vi "Actor Core.vi"(8 "error in":errorcluster, 11 "Nested in":refnum<class "TriaxesStageController.lvclass">) -> (0 "error out":errorcluster, 3 "Actor out":refnum<class "Actor.lvclass">)   [LabVIEW 2020, in "TriaxesStageController.lvlib" / "TriaxesStageController.lvclass"]
doc: "(<B>Filename</B>: Actor Framework.lvlib:Actor.lvclass:Actor Core.vi)\n\nReceives messages to the actor, reacts to them, and initiates any error handling that may shut the actor down.\n\nDescendant classes may override this VI to append parallel tasks for the actor to complete while it handles messages. Overrides use the Call Parent Method node."
uses:
  TriaxesStageController.lvclass
  C:/Program Files/National Instruments/LabVIEW 2020/vi.lib/ActorFramework/Actor/Actor.lvclass
  <vilib>/ActorFramework/Actor/Actor.lvclass
  TriaxesStageController.lvclass/TriaxesStageController.ctl
  <vilib>/ActorFramework/Actor/Actor.lvclass/Actor.ctl
  <vilib>/ActorFramework/Message Enqueuer/Message Enqueuer.lvclass/Message Enqueuer.ctl
  Model/Hardware Abstraction Layer/Component/Stage/Stage Messages/SetRelativePositionUm Msg/SetRelativePositionUm Msg.lvclass/SetRelativePositionUm Msg.ctl
  Model/Hardware Abstraction Layer/Component/Stage/Stage Messages/SetPositionUm Msg/SetPositionUm Msg.lvclass/SetPositionUm Msg.ctl
  Model/Hardware Abstraction Layer/Component/Device/Device Messages/SetSamplingRate Msg/SetSamplingRate Msg.lvclass/SetSamplingRate Msg.ctl
  <vilib>/ActorFramework/Message Enqueuer/Init from Existing Queue.vi
  <vilib>/ActorFramework/Message Enqueuer/Enqueue.vi
  Model/Hardware Abstraction Layer/Component/Stage/Stage Messages/SetRelativePositionUm Msg/SetRelativePositionUm Msg.lvclass
  C:/Program Files/National Instruments/LabVIEW 2020/vi.lib/ActorFramework/Message/Message.lvclass
  Model/Hardware Abstraction Layer/Component/Stage/Stage Messages/SetPositionUm Msg/SetPositionUm Msg.lvclass
  Model/Hardware Abstraction Layer/Component/Device/Device Messages/SetSamplingRate Msg/SetSamplingRate Msg.lvclass
  <vilib>/ActorFramework/Stop Msg/Stop Msg.lvclass
  <vilib>/ActorFramework/Message Priority Queue/Priority Enqueue.vi
  <vilib>/ActorFramework/Message Enqueuer/Message Enqueuer.lvclass
panel:
  in  "SamplingRate(Hz)":dbl min=0.0 max=200.0
  in  "Stop Button":bool
  in  "StageZ":dbl min=0.0 max=200.0
  in  "StageY":dbl min=0.0 max=200.0
  in  "StageX":dbl min=0.0 max=200.0
  out "NanoStage X":dbl(graph)
  out "NanoStage  Y":dbl(graph)
  out "NanoStage Z":dbl(graph)
  in  "ZIncreatement+":dbl min=0.0 max=50.0
  in  "ZIncreatement++":dbl min=0.0 max=50.0
  in  "StageX-":bool
  in  "StageX+":bool
  in  "StageY+":bool
  in  "StageY-":bool
  in  "StageY++":bool
  in  "StageX--":bool
  in  "StageX++":bool
  in  "StageY--":bool
  in  "XYIncreatement+":dbl min=0.0 max=50.0
  in  "XYIncreatement++":dbl min=0.0 max=100.0
  in  "StageZ++":bool
  in  "StageZ--":bool
  in  "StageZ+":bool
  in  "StageZ-":bool
  # "Increment(um)"
  # "um"
  # "um"
  # "um"
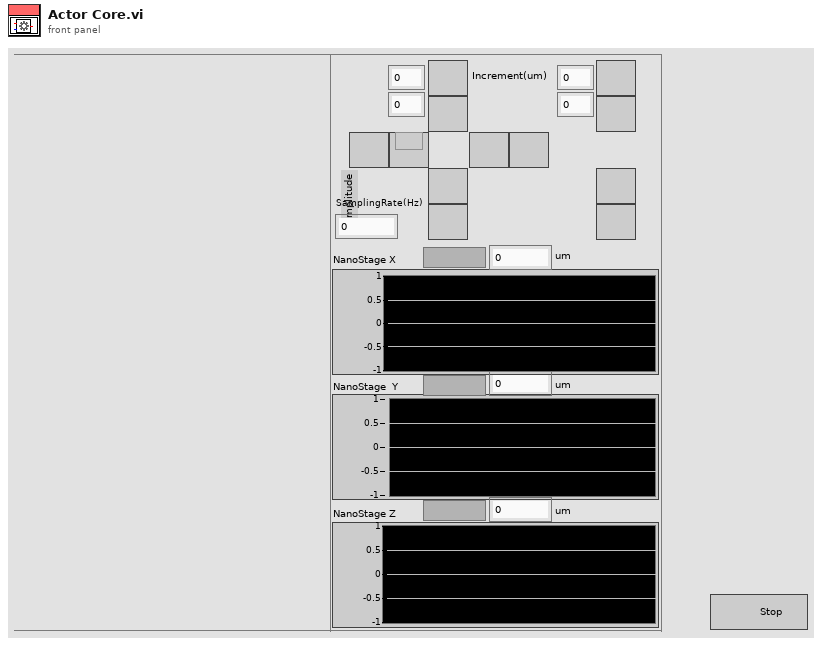
[diagram p1: front panel]
types:
  T1 = cluster{"Stop":refnum<user-event>, "NanoStage X":refnum<user-event>, "NanoStage  Y":refnum<user-event>, "NanoStage Z":refnum<user-event>}
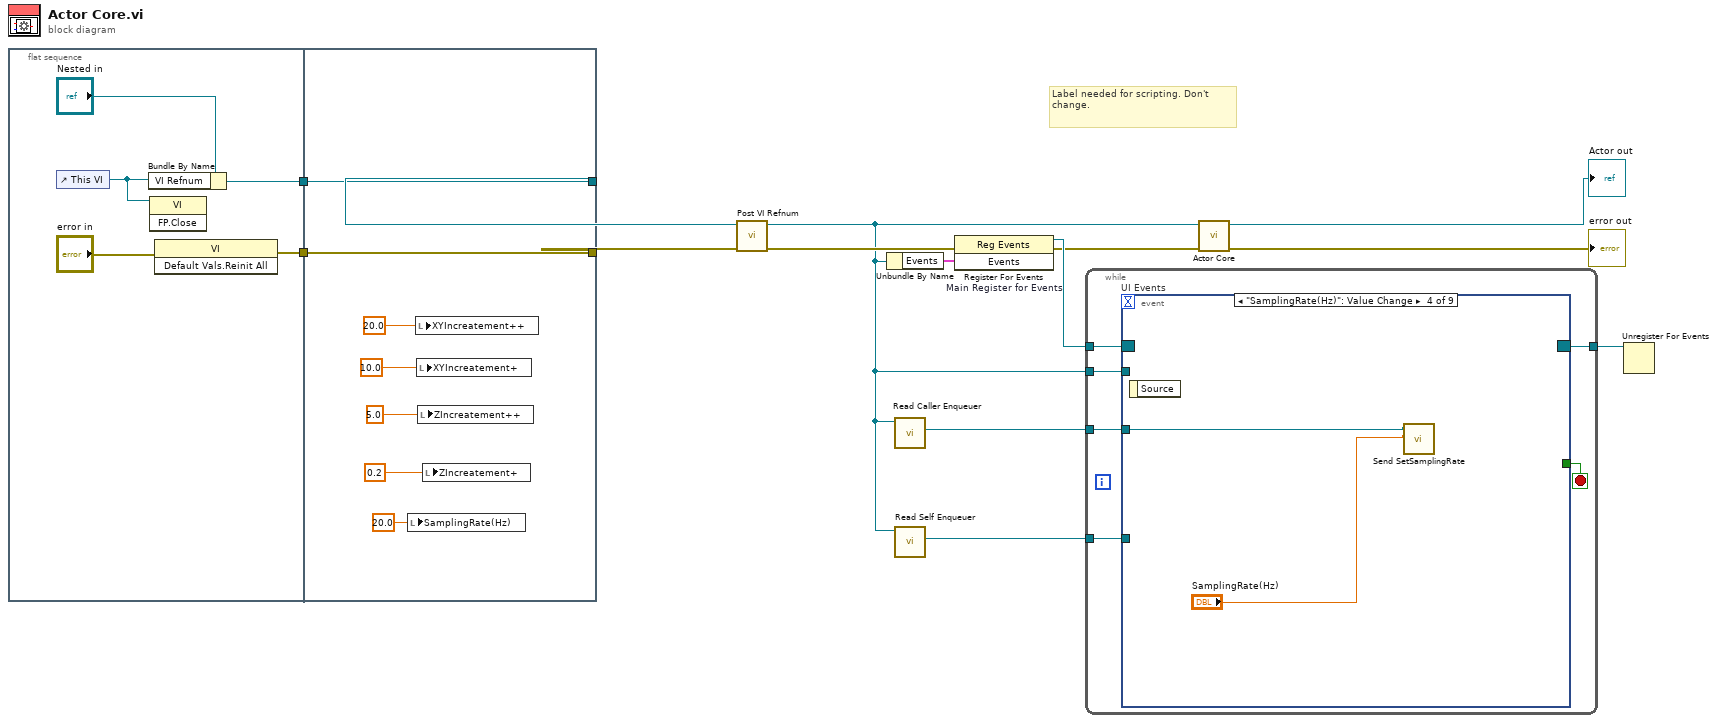
[diagram p0: block diagram]
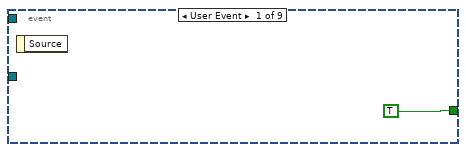
[diagram p2: hidden frame]
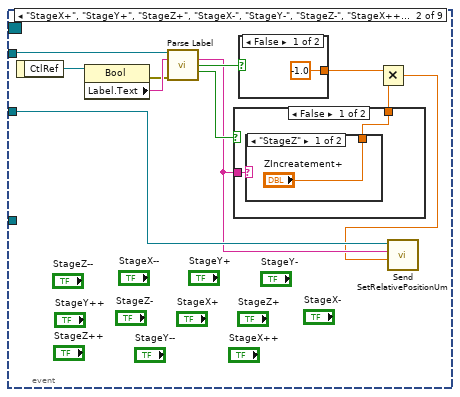
[diagram p3: hidden frame]
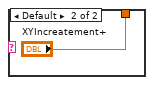
[diagram p4: hidden frame]
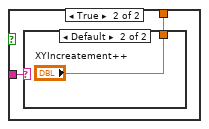
[diagram p5: hidden frame]
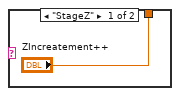
[diagram p6: hidden frame]
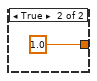
[diagram p7: hidden frame]
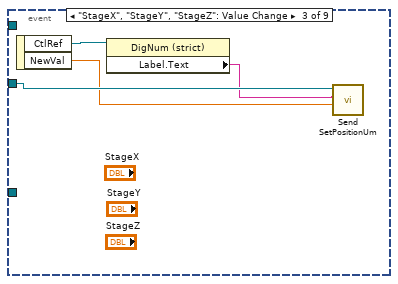
[diagram p8: hidden frame]
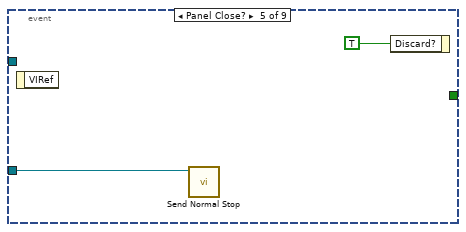
[diagram p9: hidden frame]
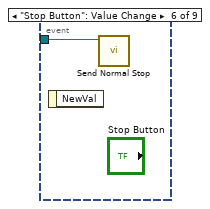
[diagram p10: hidden frame]
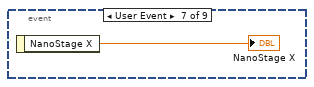
[diagram p11: hidden frame]
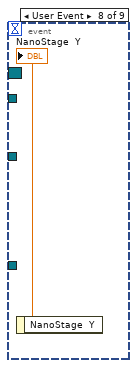
[diagram p12: hidden frame]
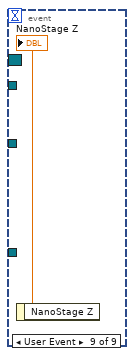
[diagram p13: hidden frame]
diagram:
  # "Label needed for scripting. Don't change."
  n1 = flat-sequence {
    tunnel: [w17] -> w2
    tunnel: [w16] -> w1
    tunnel: [w25] -> w6
    tunnel: [w26] -> w7
    tunnel: w2 -> [w26]
    tunnel: w1 -> [w25]
    frame #0 {
      n2 = control-ref of="This VI"() -> (w15:refnum<vi>)
      n3 = Bundle By Name(cluster="Nested in", "VI Refnum"=w15) -> (w17:refnum<class "TriaxesStageController.lvclass">)
      n4 = invoke class="VI" method="FP.Close"(reference=w15) -> ()  [unwired: 2 in, 3 out]
      n5 = invoke class="VI" method="Default Vals.Reinit All"(error in="error in") -> (error out=w16:errorcluster)  [unwired: 2 in, 2 out]
    }
    frame #1 {
      n6 = local write "SamplingRate(Hz)"(20.0 ("Interval(ms)")) -> ()
      n7 = local write "XYIncreatement++"(20.0 ("XYIncreatement++")) -> ()
      n8 = local write "XYIncreatement+"(10.0 ("XYIncreatement++")) -> ()
      n9 = local write "ZIncreatement++"(5.0 ("XYIncreatement++")) -> ()
      n10 = local write "ZIncreatement+"(0.2 ("XYIncreatement++")) -> ()
    }
  }
  n11 = call-dynamic "Post VI Refnum.vi"("error in (no error)"=w6, "Stage Controller in"=w7) -> ("error out"=w5:errorcluster, "Stage Controller out"=w4:refnum<class "TriaxesStageController.lvclass">)  [unwired: 8 in]
  n12 = Unbundle By Name(w4) -> ("Events"=w11:T1)
  n13 = call <vilib>:"Read Caller Enqueuer.vi"("Actor"=w4) -> ("Caller Enqueuer"=w3:refnum<class "Message Enqueuer.lvclass">)  [unwired: 10 in]
  n14 = call <vilib>:"Read Self Enqueuer.vi"("Actor"=w4) -> ("Self Enqueuer"=w9:refnum<class "Message Enqueuer.lvclass">)  [unwired: 10 in]
  n15 = register-events "Main Register for Events"(error in=w5, w11) -> (reference out=w12:refnum<event-registration>, error out=w8:errorcluster)  [unwired: 1 in]
  n16 = while {
    tunnel: w12 -> [w32]
    tunnel: [w30] -> w10
    tunnel: w9 -> [w29]
    tunnel: w4 -> [w28]
    tunnel: w3 -> [w27]
    stop <- w31 stop-if-true
    n17 = event "UI Events" shown="[3] \"SamplingRate(Hz)\": Value Change" {
      selector: w32 -> [_ _ _ _ _ _ _ _ _]
      dyn-events: [_ _ _ _ _ _ _ _ _] -> w30
      timeout: _ -> [_ _ _ _ _ _ _ _ _]
      tunnel: [TRUE _ _ _ _ _ _ _ _] -> w31
      tunnel: w29 -> [_ _ _ _ w61 w63 _ _ _]
      tunnel: w28 -> [_ w41 _ _ _ _ _ _ _]
      tunnel: w27 -> [_ w36 w57 w60 _ _ _ _ _]
      event User Event {
        n18 = event-data() -> ()  [unwired: 1 in, 1 out]
      }
      event "StageX+", "StageY+", "StageZ+", "StageX-", "StageY-", "StageZ-", "StageX++", "StageY++", "StageZ++", "StageX--", "StageY--", "StageZ--": Value Change {
        n19 = event-data() -> ("CtlRef"=w44:refnum<vi>)  [unwired: 1 in]
        n20 = property class="Bool"(reference=w44) -> (error out=w42:errorcluster, "Label.Text"=w43:string)  [unwired: 1 in, 1 out]
        n21 = call-dynamic "Parse Label.vi"("Stage Controller in"=w41, "Label.Text"=w43, "error in (no error)"=w42) -> ("Stage Label"=w35:string, "Increase?"=w40:bool, "Big Step?"=w39:bool)  [unwired: 8 in, 2 out]
        n22 = case shown="False" w39 {
          tunnel: [w46 w50] -> w37
          tunnel: w35 -> [w45 w49]
          frame False {
            n23 = case shown="\"StageZ\"" w45 {
              tunnel: ["ZIncreatement+" "XYIncreatement+"] -> w46
              frame "StageZ" {
              }
              frame Default {
              }
            }
          }
          frame True {
            n24 = case shown="Default" w49 {
              tunnel: ["ZIncreatement++" "XYIncreatement++"] -> w50
              frame "StageZ" {
              }
              frame Default {
              }
            }
          }
        }
        n25 = case shown="False" w40 {
          tunnel: [-1.0 ("XYIncreatement+") 1.0 ("XYIncreatement+")] -> w38
          frame False {
          }
          frame True {
          }
        }
        n26 = Multiply(x=w38, y=w37) -> (x*y=w34:dbl)
        n27 = call "Send SetRelativePositionUm.vi"("RelativeMoveum"=w34, "Stage Label"=w35, "Message Enqueuer"=w36) -> ()  [unwired: 7 in, 2 out]
      }
      event "StageX", "StageY", "StageZ": Value Change {
        n28 = event-data() -> ("CtlRef"=w58:refnum<vi>, "NewVal"=w55:dbl)  [unwired: 1 in]
        n29 = property class="DigNum (strict)"(reference=w58) -> ("Label.Text"=w56:string)  [unwired: 1 in, 2 out]
        n30 = call "Send SetPositionUm.vi"("Positionum"=w55, "Stage Label"=w56, "Message Enqueuer"=w57) -> ()  [unwired: 7 in, 2 out]
      }
      event "SamplingRate(Hz)": Value Change {
        n31 = event-data() -> ()  [unwired: 1 in, 1 out]
        n32 = call "Send SetSamplingRate.vi"("SamplingRate"="SamplingRate(Hz)", "Message Enqueuer"=w60) -> ()  [unwired: 8 in, 2 out]
      }
      event Panel Close? {
        n33 = event-data() -> ()  [unwired: 1 in, 1 out]
        n34 = call <vilib>:"Send Normal Stop.vi"("Message Enqueuer"=w61) -> ()  [unwired: 10 in, 1 out]
        n35 = event-data("Discard?"=TRUE) -> ()  [unwired: 1 in, 1 out]
      }
      event "Stop Button": Value Change {
        n36 = event-data() -> ()  [unwired: 1 in, 1 out]
        n37 = call <vilib>:"Send Normal Stop.vi"("Message Enqueuer"=w63) -> ()  [unwired: 10 in, 1 out]
      }
      event User Event {
        n38 = event-data() -> ("NanoStage X"=→"NanoStage X":dbl)  [unwired: 1 in]
      }
      event User Event {
        n39 = event-data() -> ("NanoStage  Y"=→"NanoStage  Y":dbl)  [unwired: 1 in]
      }
      event User Event {
        n40 = event-data() -> ("NanoStage Z"=→"NanoStage Z":dbl)  [unwired: 1 in]
      }
    }
  }
  n41 = call-parent "Actor Core.vi"("error in"=w8, "Actor in"=w4) -> ("error out"=→"error out":errorcluster, "Actor out"=→"Actor out":refnum<class "Actor.lvclass">)  [unwired: 8 in]
  n42 = Unregister For Events(event registration refnum=w10) -> ()  [unwired: 1 in, 1 out]
